vi "Logdata (SubVI).vi"(0 "Signals out":dbl[](array[numeric]), 1 "Ship pos":dbl[](array[numeric]), 5 "MT_DATA":dbl[](array[numeric]), 7 "Vessel in":refnum<class "Vessel.lvclass">, 9 "dvl_m":dbl[](array[numeric]), 11 "error in (no error)":errorcluster, 12 "MT_BITS":u8[](array[numeric]), 14 "kPa":dbl) -> (15 "error out":errorcluster)   [LabVIEW 2012]
uses:
  ROV/Vessel.lvclass
panel:
  out "log line tau":string="21:11:09.2343\t-0.00\t0.00\t30.00\t0.00\t0.00\t-0.00\t0.00\t0.01\t-0.01\t-0.00\t30.00\t0.00\t0.00\t-0.00\t0.00\t0.00\t0.00\t0.00\t30.00\t0.00\t0.00\t0.00\t0.00\t0.00\t132.54\t-43.98\t11.70\t-0.09\t-661 \t252 \t818 \t705 \r\n"
  out "log line nu":string="21:11:09.2343\t-0.00\t0.00\t30.00\t0.00\t0.00\t-0.00\t0.00\t0.01\t-0.01\t-0.00\t30.00\t0.00\t0.00\t-0.00\t0.00\t0.00\t0.00\t0.00\t30.00\t0.00\t0.00\t0.00\t0.00\t0.00\t132.54\t-43.98\t11.70\t-0.09\t-661 \t252 \t818 \t705 \r\n"
  out "log line eta":string="21:11:09.2343\t-0.00\t0.00\t30.00\t0.00\t0.00\t-0.00\t0.00\t0.01\t-0.01\t-0.00\t30.00\t0.00\t0.00\t-0.00\t0.00\t0.00\t0.00\t0.00\t30.00\t0.00\t0.00\t0.00\t0.00\t0.00\t132.54\t-43.98\t11.70\t-0.09\t-661 \t252 \t818 \t705 \r\n"
  out "log line raw":string="21:11:09.2343\t-0.00\t0.00\t30.00\t0.00\t0.00\t-0.00\t0.00\t0.01\t-0.01\t-0.00\t30.00\t0.00\t0.00\t-0.00\t0.00\t0.00\t0.00\t0.00\t30.00\t0.00\t0.00\t0.00\t0.00\t0.00\t132.54\t-43.98\t11.70\t-0.09\t-661 \t252 \t818 \t705 \r\n"
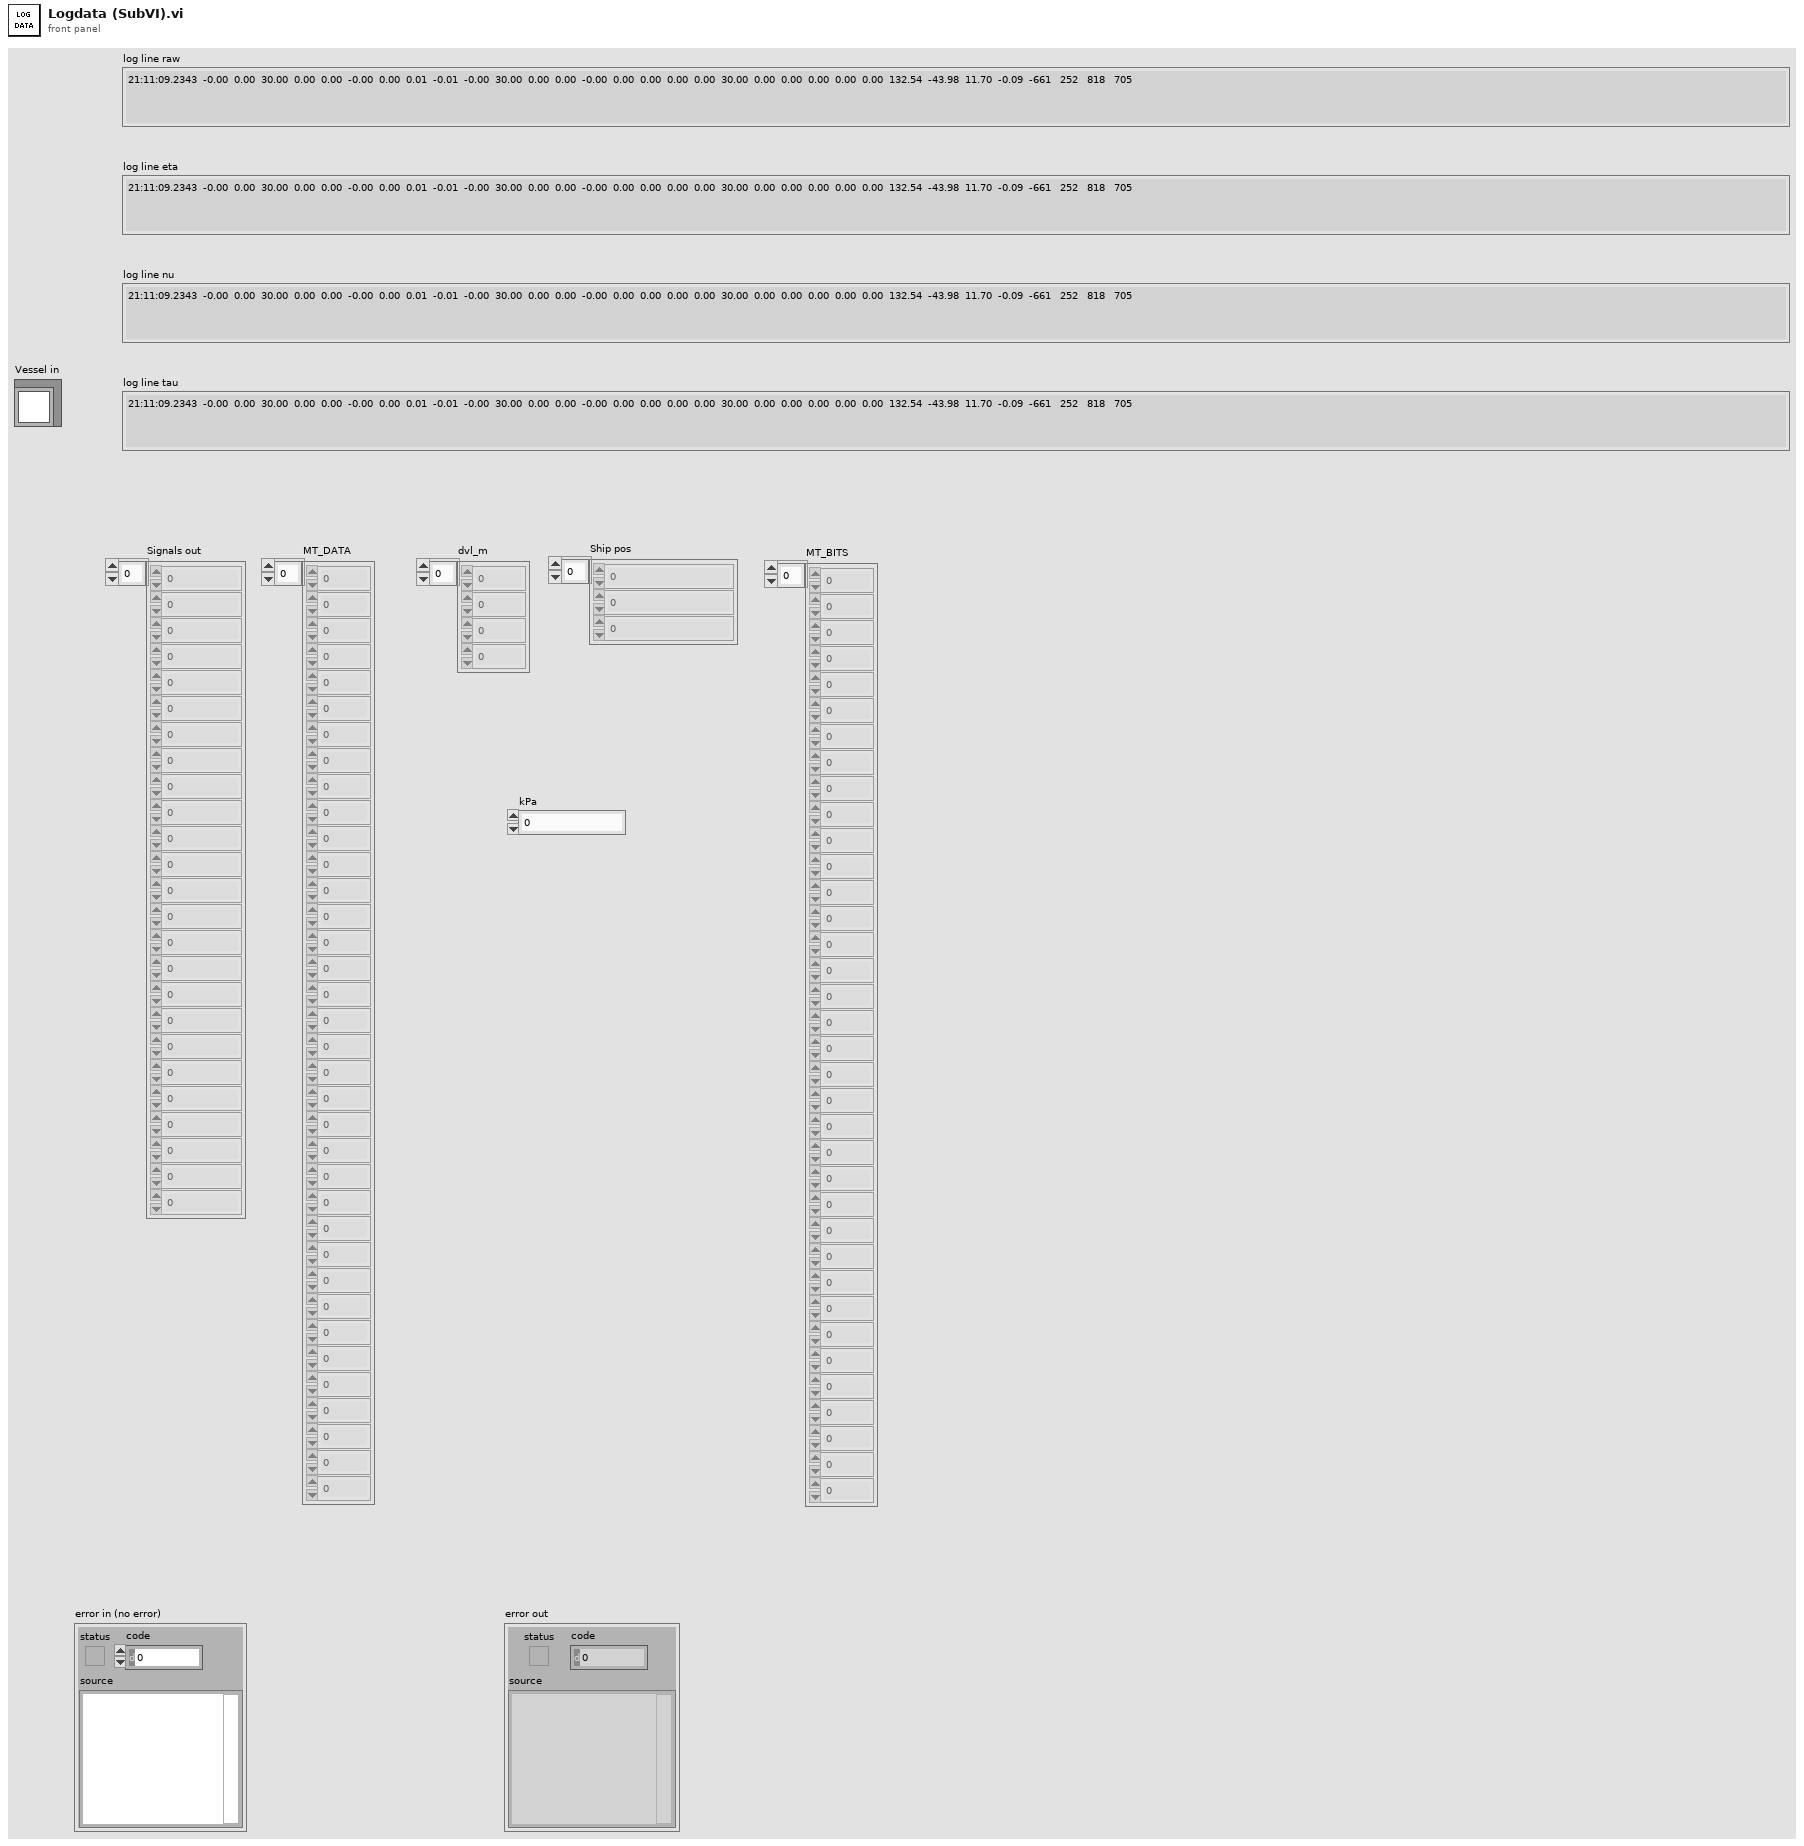
[diagram p1: front panel]
types:
  T1 = cluster{"Measured":cluster{"Eta":dbl[], "Nu":dbl[], "Eta Dot":dbl[], "Nu Dot":dbl[]}, "Estimated":cluster{"Eta":dbl[], "Nu":dbl[], "Eta Dot":dbl[], "Nu Dot":dbl[]}, "Desired":cluster{"Eta":dbl[], "Nu":dbl[], "Eta Dot":dbl[], "Nu Dot":dbl[]}, "Previous Desired":cluster{"Eta":dbl[], "Nu":dbl[], "Eta Dot":dbl[], "Nu Dot":dbl[]}, "tau":dbl[], "Altitude":cluster{"Measured":dbl, "Estimated":dbl, "Desired":dbl, "Previous Desired":dbl, "Approximated":dbl, "grad F":dbl[]}, "rpm":dbl[], "Attitude":cluster{"Theta Measured":dbl[], "Theta Estimated":dbl[], "Omega Measured":dbl[], "Omega Estimated":dbl[]}}
  T2 = enum16{"open", "replace", "create", "open or create", "replace or create", "replace or create with confirmation"}
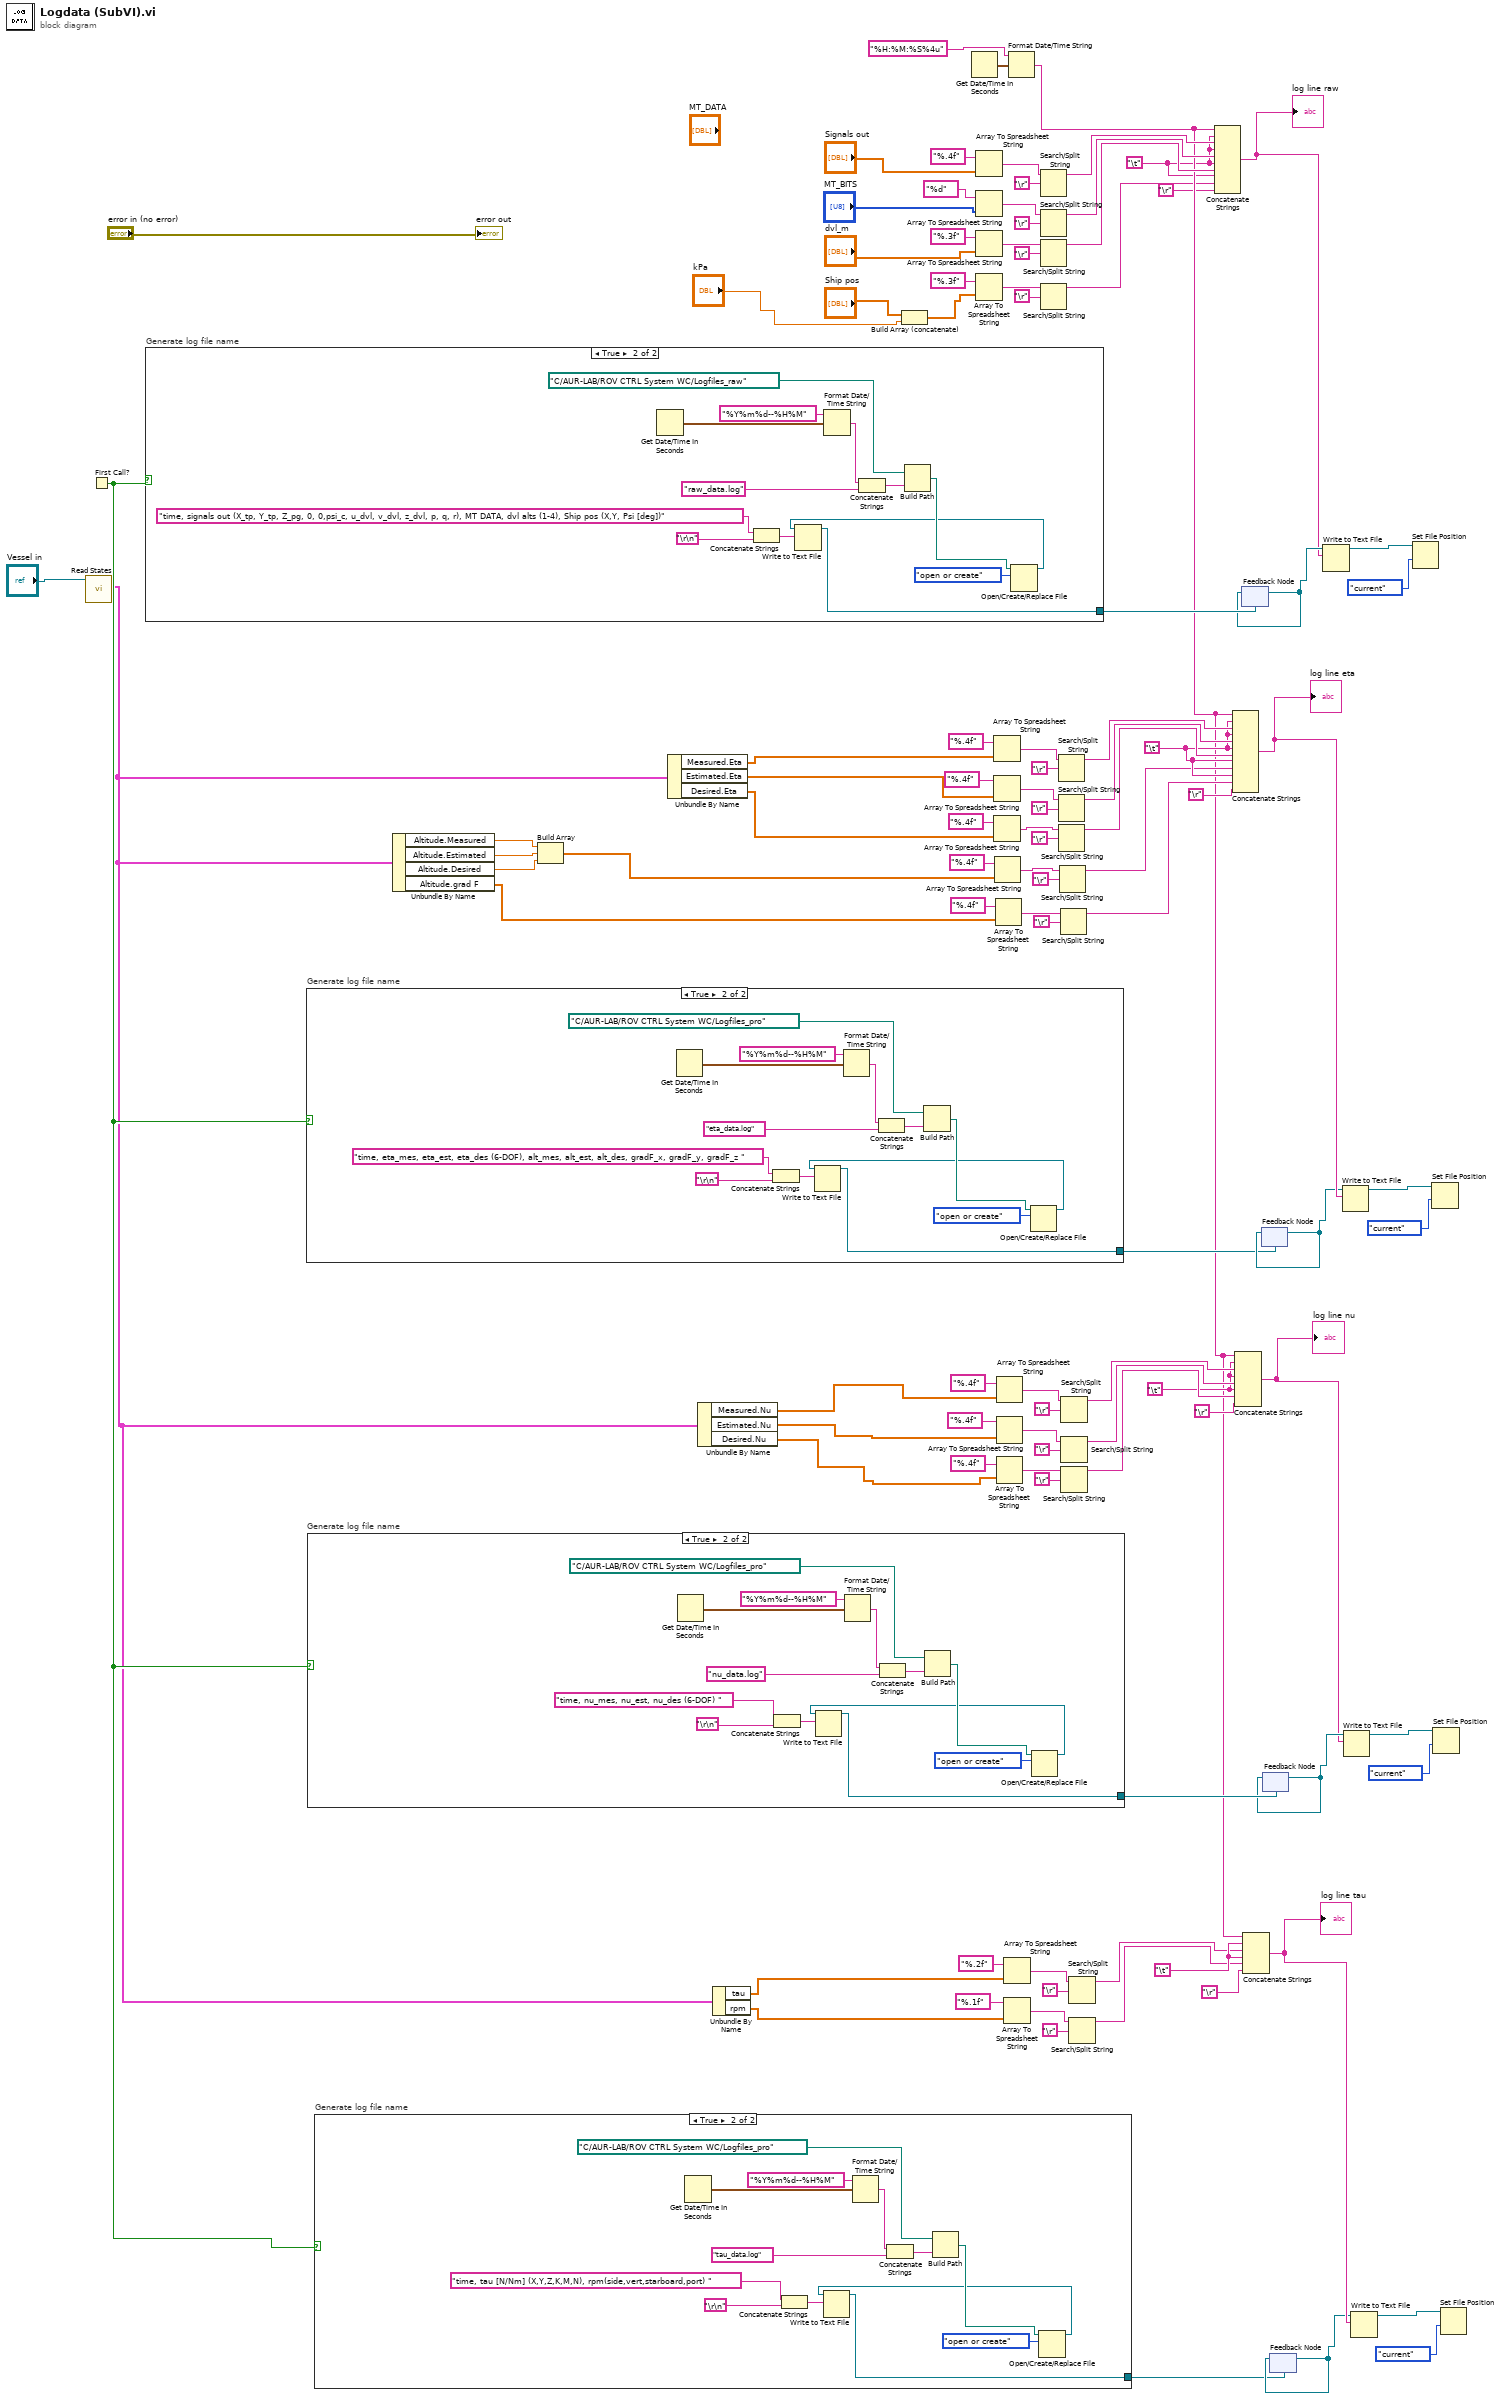
[diagram p0: block diagram]
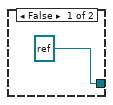
[diagram p2: hidden frame]
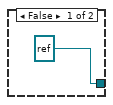
[diagram p3: hidden frame]
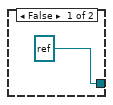
[diagram p4: hidden frame]
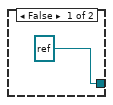
[diagram p5: hidden frame]
diagram:
  w26 = "\t"
  w58 = "\t"
  w43 = "\t"
  w8 = "\t"
  n1 = call-dynamic "Read States.vi"("Vessel in"="Vessel in") -> ("States"=w14:T1)  [unwired: 8 in, 2 out]
  n2 = First Call?() -> (First Call?: T/F=w15:bool)
  n3 = case "Generate log file name" shown="True" w15 {
    tunnel: [refnum<file> refnum ("refnum out") w112] -> w97
    frame False {
    }
    frame True {
      n4 = Get Date/Time In Seconds() -> (seconds since 1Jan1904=w120:timestamp)
      n5 = Concatenate Strings("time, signals out (X_tp, Y_tp, Z_pg, 0, 0,psi_c, u_dvl, v_dvl, z_dvl, p, q, r), MT DATA, dvl alts (1-4), Ship pos (X,Y, Psi [deg])" ("string"), "\r\n") -> (w114:string)
      n6 = Format Date/Time String(time format string (%c)="%Y%m%d--%H%M", seconds (now)=w120) -> (date/time string=w118:string)  [unwired: 1 in]
      n7 = Concatenate Strings(w118, "raw_data.log" ("string")) -> (w123:string)
      n8 = Build Path(base path=path "C:/AUR-LAB/ROV CTRL System WC/Logfiles_raw" ("file path (use dialog)"), name or relative path=w123) -> (appended path=w121:path)
      n9 = Open/Create/Replace File(file path (use dialog)=w121, operation (0:open)=T2."open or create") -> (refnum out=w113:refnum<file>)  [unwired: 4 in, 2 out]
      n10 = Write to Text File(file (use dialog)=w113, text=w114) -> (refnum out=w112:refnum<file>)  [unwired: 2 in, 2 out]
    }
  }
  n11 = case "Generate log file name" shown="True" w15 {
    tunnel: [refnum<file> refnum ("refnum out") w126] -> w84
    frame False {
    }
    frame True {
      n12 = Get Date/Time In Seconds() -> (seconds since 1Jan1904=w134:timestamp)
      n13 = Concatenate Strings("time, eta_mes, eta_est, eta_des (6-DOF), alt_mes, alt_est, alt_des, gradF_x, gradF_y, gradF_z " ("string"), "\r\n") -> (w128:string)
      n14 = Format Date/Time String(time format string (%c)="%Y%m%d--%H%M", seconds (now)=w134) -> (date/time string=w132:string)  [unwired: 1 in]
      n15 = Concatenate Strings(w132, "eta_data.log" ("string")) -> (w137:string)
      n16 = Build Path(base path=path "C:/AUR-LAB/ROV CTRL System WC/Logfiles_pro" ("file path (use dialog)"), name or relative path=w137) -> (appended path=w135:path)
      n17 = Open/Create/Replace File(file path (use dialog)=w135, operation (0:open)=T2."open or create") -> (refnum out=w127:refnum<file>)  [unwired: 4 in, 2 out]
      n18 = Write to Text File(file (use dialog)=w127, text=w128) -> (refnum out=w126:refnum<file>)  [unwired: 2 in, 2 out]
    }
  }
  n19 = case "Generate log file name" shown="True" w15 {
    tunnel: [refnum<file> refnum ("refnum out") w141] -> w60
    frame False {
    }
    frame True {
      n20 = Get Date/Time In Seconds() -> (seconds since 1Jan1904=w148:timestamp)
      n21 = Concatenate Strings("time, nu_mes, nu_est, nu_des (6-DOF) " ("string"), "\r\n") -> (w143:string)
      n22 = Format Date/Time String(time format string (%c)="%Y%m%d--%H%M", seconds (now)=w148) -> (date/time string=w146:string)  [unwired: 1 in]
      n23 = Concatenate Strings(w146, "nu_data.log" ("string")) -> (w151:string)
      n24 = Build Path(base path=path "C:/AUR-LAB/ROV CTRL System WC/Logfiles_pro" ("file path (use dialog)"), name or relative path=w151) -> (appended path=w149:path)
      n25 = Open/Create/Replace File(file path (use dialog)=w149, operation (0:open)=T2."open or create") -> (refnum out=w142:refnum<file>)  [unwired: 4 in, 2 out]
      n26 = Write to Text File(file (use dialog)=w142, text=w143) -> (refnum out=w141:refnum<file>)  [unwired: 2 in, 2 out]
    }
  }
  n27 = case "Generate log file name" shown="True" w15 {
    tunnel: [refnum<file> refnum ("refnum out") w155] -> w24
    frame False {
    }
    frame True {
      n28 = Get Date/Time In Seconds() -> (seconds since 1Jan1904=w162:timestamp)
      n29 = Concatenate Strings("time, tau [N/Nm] (X,Y,Z,K,M,N), rpm(side,vert,starboard,port) " ("string"), "\r\n") -> (w157:string)
      n30 = Format Date/Time String(time format string (%c)="%Y%m%d--%H%M", seconds (now)=w162) -> (date/time string=w160:string)  [unwired: 1 in]
      n31 = Concatenate Strings(w160, "tau_data.log" ("string")) -> (w165:string)
      n32 = Build Path(base path=path "C:/AUR-LAB/ROV CTRL System WC/Logfiles_pro" ("file path (use dialog)"), name or relative path=w165) -> (appended path=w163:path)
      n33 = Open/Create/Replace File(file path (use dialog)=w163, operation (0:open)=T2."open or create") -> (refnum out=w156:refnum<file>)  [unwired: 4 in, 2 out]
      n34 = Write to Text File(file (use dialog)=w156, text=w157) -> (refnum out=w155:refnum<file>)  [unwired: 2 in, 2 out]
    }
  }
  n35 = Unbundle By Name(w14) -> ("Altitude.Measured"=w46:dbl, "Altitude.Estimated"=w45:dbl, "Altitude.Desired"=w44:dbl, "Altitude.grad F"=w33:dbl[])
  n36 = Build Array(w46, w45, w44) -> (w39:dbl[])
  n37 = Unbundle By Name(w14) -> ("Measured.Eta"=w52:dbl[], "Estimated.Eta"=w51:dbl[], "Desired.Eta"=w50:dbl[])
  n38 = Unbundle By Name(w14) -> ("Measured.Nu"=w49:dbl[], "Estimated.Nu"=w48:dbl[], "Desired.Nu"=w47:dbl[])
  n39 = Unbundle By Name(w14) -> ("tau"=w30:dbl[], "rpm"=w31:dbl[])
  n40 = Build Array (concatenate)("Ship pos", "kPa") -> (w3:dbl[])
  n41 = Get Date/Time In Seconds() -> (seconds since 1Jan1904=w100:timestamp)
  n42 = Array To Spreadsheet String(array="Signals out", 3:"%.4f" ("format string")) -> (spreadsheet string=w91:string)  [unwired: 1 in]
  n43 = Array To Spreadsheet String(array="MT_BITS", 3:"%d" ("format string")) -> (spreadsheet string=w90:string)  [unwired: 1 in]
  n44 = Array To Spreadsheet String(array="dvl_m", 3:"%.3f" ("format string")) -> (spreadsheet string=w106:string)  [unwired: 1 in]
  n45 = Array To Spreadsheet String(array=w3, 3:"%.3f" ("format string")) -> (spreadsheet string=w11:string)  [unwired: 1 in]
  n46 = Array To Spreadsheet String(array=w52, 3:"%.4f" ("format string")) -> (spreadsheet string=w88:string)  [unwired: 1 in]
  n47 = Array To Spreadsheet String(array=w51, 3:"%.4f" ("format string")) -> (spreadsheet string=w89:string)  [unwired: 1 in]
  n48 = Array To Spreadsheet String(array=w50, 3:"%.4f" ("format string")) -> (spreadsheet string=w41:string)  [unwired: 1 in]
  n49 = Array To Spreadsheet String(array=w39, 3:"%.4f" ("format string")) -> (spreadsheet string=w34:string)  [unwired: 1 in]
  n50 = Array To Spreadsheet String(array=w33, 3:"%.4f" ("format string")) -> (spreadsheet string=w36:string)  [unwired: 1 in]
  n51 = Array To Spreadsheet String(array=w49, 3:"%.4f" ("format string")) -> (spreadsheet string=w55:string)  [unwired: 1 in]
  n52 = Array To Spreadsheet String(array=w48, 3:"%.4f" ("format string")) -> (spreadsheet string=w54:string)  [unwired: 1 in]
  n53 = Array To Spreadsheet String(array=w47, 3:"%.4f" ("format string")) -> (spreadsheet string=w67:string)  [unwired: 1 in]
  n54 = Array To Spreadsheet String(array=w30, 3:"%.2f" ("format string")) -> (spreadsheet string=w28:string)  [unwired: 1 in]
  n55 = Array To Spreadsheet String(array=w31, 3:"%.1f" ("format string")) -> (spreadsheet string=w29:string)  [unwired: 1 in]
  n56 = Format Date/Time String(time format string (%c)="%H:%M:%S%4u", seconds (now)=w100) -> (date/time string=w12:string)  [unwired: 1 in]
  n57 = Search/Split String(string=w91, search string/char (-)="\r") -> (substring before match=w105:string)  [unwired: 1 in, 2 out]
  n58 = Search/Split String(string=w90, search string/char (-)="\r") -> (substring before match=w104:string)  [unwired: 1 in, 2 out]
  n59 = Search/Split String(string=w106, search string/char (-)="\r") -> (substring before match=w103:string)  [unwired: 1 in, 2 out]
  n60 = Search/Split String(string=w11, search string/char (-)="\r") -> (substring before match=w7:string)  [unwired: 1 in, 2 out]
  n61 = Search/Split String(string=w88, search string/char (-)="\r") -> (substring before match=w78:string)  [unwired: 1 in, 2 out]
  n62 = Search/Split String(string=w89, search string/char (-)="\r") -> (substring before match=w79:string)  [unwired: 1 in, 2 out]
  n63 = Search/Split String(string=w41, search string/char (-)="\r") -> (substring before match=w80:string)  [unwired: 1 in, 2 out]
  n64 = Search/Split String(string=w34, search string/char (-)="\r") -> (substring before match=w38:string)  [unwired: 1 in, 2 out]
  n65 = Search/Split String(string=w36, search string/char (-)="\r") -> (substring before match=w32:string)  [unwired: 1 in, 2 out]
  n66 = Search/Split String(string=w55, search string/char (-)="\r") -> (substring before match=w66:string)  [unwired: 1 in, 2 out]
  n67 = Search/Split String(string=w54, search string/char (-)="\r") -> (substring before match=w65:string)  [unwired: 1 in, 2 out]
  n68 = Search/Split String(string=w67, search string/char (-)="\r") -> (substring before match=w64:string)  [unwired: 1 in, 2 out]
  n69 = Search/Split String(string=w28, search string/char (-)="\r") -> (substring before match=w20:string)  [unwired: 1 in, 2 out]
  n70 = Search/Split String(string=w29, search string/char (-)="\r") -> (substring before match=w21:string)  [unwired: 1 in, 2 out]
  n71 = Concatenate Strings(w12, w8, w105, w8, w104, w8, w103, w8, w7, "\r") -> (w93:string)
  "log line raw" <- w93
  n72 = Concatenate Strings(w12, w43, w78, w43, w79, w43, w80, w43, w38, w43, w32, "\r") -> (w87:string)
  "log line eta" <- w87
  n73 = Concatenate Strings(w12, w58, w66, w58, w65, w58, w64, "\r") -> (w56:string)
  "log line nu" <- w56
  n74 = feedback #1(w97) -> (w96:refnum<file>)
  n75 = feedback-in #1(w96) -> ()
  n76 = Concatenate Strings(w12, w26, w20, w26, w21, "\r") -> (w27:string)
  "log line tau" <- w27
  n77 = feedback #2(w84) -> (w85:refnum<file>)
  n78 = feedback-in #2(w85) -> ()
  n79 = feedback #3(w60) -> (w59:refnum<file>)
  n80 = feedback-in #3(w59) -> ()
  n81 = feedback #4(w24) -> (w25:refnum<file>)
  n82 = feedback-in #4(w25) -> ()
  n83 = Write to Text File(file (use dialog)=w96, text=w93) -> (refnum out=w99:refnum<file>)  [unwired: 2 in, 2 out]
  n84 = Write to Text File(file (use dialog)=w85, text=w87) -> (refnum out=w82:refnum<file>)  [unwired: 2 in, 2 out]
  n85 = Write to Text File(file (use dialog)=w59, text=w56) -> (refnum out=w62:refnum<file>)  [unwired: 2 in, 2 out]
  n86 = Write to Text File(file (use dialog)=w25, text=w27) -> (refnum out=w22:refnum<file>)  [unwired: 2 in, 2 out]
  n87 = Set File Position(refnum=w99, from (0:start)=enum16{"start", "end", "current"}."current") -> ()  [unwired: 2 in, 2 out]
  n88 = Set File Position(refnum=w82, from (0:start)=enum16{"start", "end", "current"}."current") -> ()  [unwired: 2 in, 2 out]
  n89 = Set File Position(refnum=w62, from (0:start)=enum16{"start", "end", "current"}."current") -> ()  [unwired: 2 in, 2 out]
  n90 = Set File Position(refnum=w22, from (0:start)=enum16{"start", "end", "current"}."current") -> ()  [unwired: 2 in, 2 out]
  "error out" <- "error in (no error)"
